vi "Signature_Format_Save n Print Word Report (SubVI) Mult.vi"(7 "מפעיל":string="ANS", 8 "error in (no error)":errorcluster, 9 "עבר/נכשל":string="עבר/נכשל", 10 "Path":path, 11 "NI_report in":refnum<class "NI_report.lvclass">) -> (0 "error out":errorcluster)   [LabVIEW 2015]
uses:
  <vilib>/Utility/NIReport.llb/NI_report.lvclass
  <vilib>/Utility/NIReport.llb/Append Report Text (str wrap).vi
  <vilib>/Utility/NIReport.llb/Word/NI_Word.lvclass
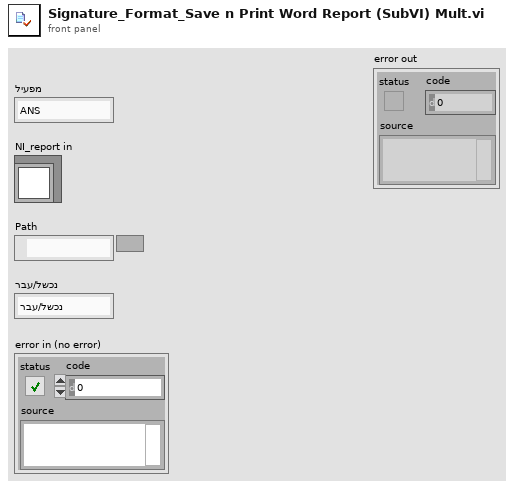
[diagram p1: front panel]
types:
  T1 = cluster{"alignment":enum16{"Left", "Centered", "Right", "Justify"}, "left":dbl, "right":dbl, "special":enum16{"(none)", "First line", "Hanging"}, "by":dbl, "before":dbl, "after":dbl, "line spacing":enum16{"Single", "1,5 lines", "Double", "At least", "Exactly", "Multiple"}, "at":dbl}
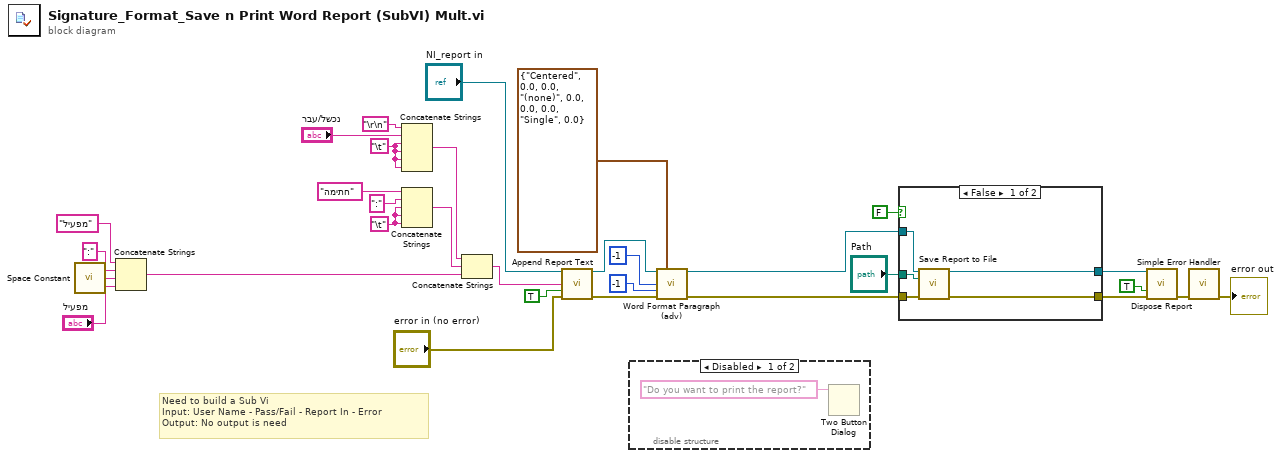
[diagram p0: block diagram]
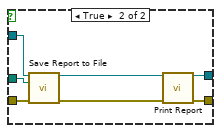
[diagram p3: hidden frame]
diagram:
  w26 = "\t"
  w1 = "\t"
  # "Need to build a Sub Vi\nInput: User Name - Pass/Fail - Report In - Error\nOutput: No output is need"
  n1 = call <vilib>:"Space Constant.vi"() -> ("String"=w3:string)
  n2 = Concatenate Strings("מפעיל" ("string"), ":" ("string"), w3, "מפעיל") -> (w22:string)
  n3 = Concatenate Strings("\r\n", "עבר/נכשל", w26, w26, w26, w26) -> (w25:string)
  n4 = Concatenate Strings("חתימה" ("string"), ":" ("string"), w1, w1, w1) -> (w21:string)
  n5 = Concatenate Strings(w25, w21, w22) -> (w23:string)
  n6 = call-poly <vilib>:"Append Report Text.vi"("report in"="NI_report in", "text"=w23, "append on new line? (F)"=TRUE, "error in (no error)"="error in (no error)") -> ("report out"=w18:refnum<class "NI_report.lvclass">, "error out"=w17:errorcluster)  [unwired: 8 in, 2 out]
  n7 = disable-structure shown="Disabled" {
    frame Disabled {
      n8 = Two Button Dialog(message="Do you want to print the report?") -> ()  [unwired: 2 in, 1 out]
    }
    frame Enabled {
    }
  }
  n9 = call <vilib>:"Word Format Paragraph (adv).vi"("report in"=w18, "indent and spacing"=T1 {"alignment"=enum."Centered", "left"=0.0, "right"=0.0, "special"=enum."(none)", "by"=0.0, "before"=0.0, "after"=0.0, "line spacing"=enum."Single", "at"=0.0}, "start (-1)"=-1, "end (-1)"=-1, "error in (no error)"=w17) -> ("report out"=w13:refnum<class "NI_report.lvclass">, "error out"=w12:errorcluster)  [unwired: 9 in]
  n10 = case shown="False" FALSE {
    tunnel: [w37 w43] -> w15
    tunnel: "Path" -> [w36 w44]
    tunnel: [w35 w41] -> w10
    tunnel: w13 -> [w34 w39]
    tunnel: w12 -> [w33 w38]
    frame False {
      n11 = call-dynamic "Save Report to File.vi"("report in"=w34, "report file path"=w36, "error in (no error)"=w33) -> ("report out"=w35:refnum<class "NI_report.lvclass">, "error out"=w37:errorcluster)  [unwired: 11 in]
    }
    frame True {
      n12 = call-dynamic "Save Report to File.vi"("report in"=w39, "report file path"=w44, "error in (no error)"=w38) -> ("report out"=w42:refnum<class "NI_report.lvclass">, "error out"=w40:errorcluster)  [unwired: 11 in]
      n13 = call-dynamic "Print Report.vi"("report in"=w42, "error in (no error)"=w40) -> ("report out"=w41:refnum<class "NI_report.lvclass">, "error out"=w43:errorcluster)  [unwired: 12 in]
    }
  }
  n14 = call-dynamic "Dispose Report.vi"("report in"=w10, "save changes? (F)"=TRUE, "error in (no error)"=w15) -> ("error out"=w16:errorcluster)  [unwired: 12 in]
  n15 = call <vilib>:"Simple Error Handler.vi"("error in (no error)"=w16) -> ("error out"=→"error out":errorcluster)  [unwired: 4 in, 4 out]
